vi "HTL_ErrorHandler.vi"(6 "error in":errorcluster) -> (0 "error out":errorcluster, 3 "All-Quit":bool)   [LabVIEW 2020]
doc: "Resets the CCD camera controller and initializes it with Setup String. The default Setup String is \"ldb,1,16,u,0,225,25,b,1,15;sdu,0,1024,1024;cl0;omrm;sron\". \nError, if no -1, is set as 0 if a serial poll detects an error (bit 15 in status bit set)\n\nSet the CCD Setup String Global variable after the command is complete."
uses:
  <vilib>/Utility/error.llb/DialogType.ctl
  Globals and TypeDefs/Type Definitions.llb/3 way Status.ctl
  Globals and TypeDefs/gDetector.vi
  Globals and TypeDefs/gSpectrometer.vi
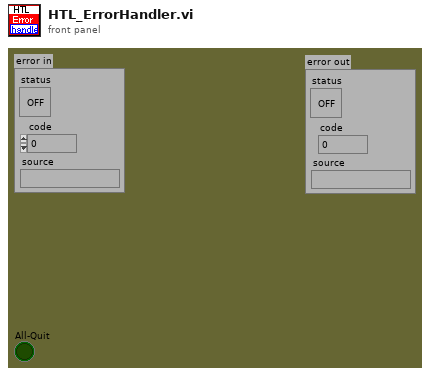
[diagram p1: front panel]
types:
  T1 = typedef "DialogType.ctl" = u16
  T2 = typedef "Error Categories.ctt" = enum8{"General", "CCD-256x1024", "CCD-1340x400", "InGaAs PDA", "McPherson 2075", "Magnetic Field", "Temperature Control", "Other"}
  T3 = enum16{"Left Button", "Center Button", "Right Button", "Window Close"}
  T4 = typedef "3 way Status.ctl" = u8
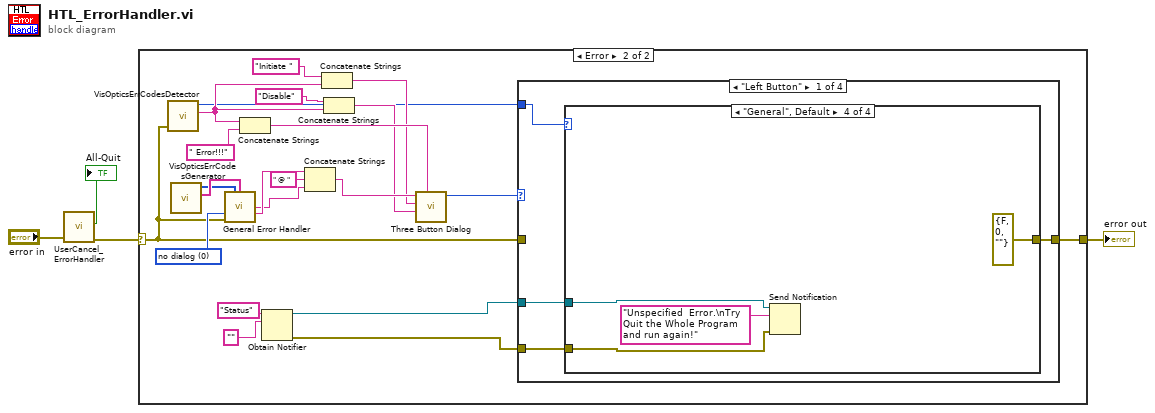
[diagram p0: block diagram]
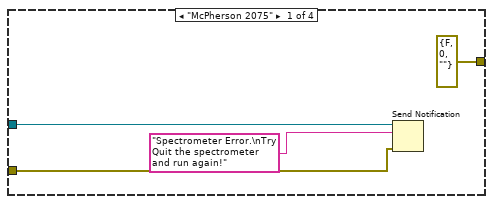
[diagram p3: hidden frame]
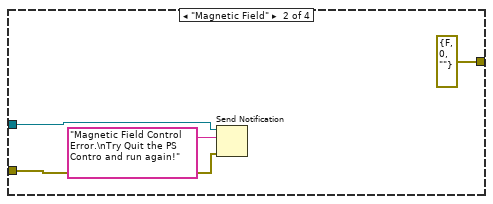
[diagram p4: hidden frame]
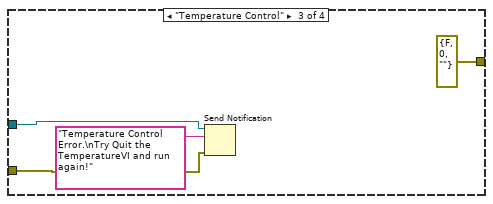
[diagram p5: hidden frame]
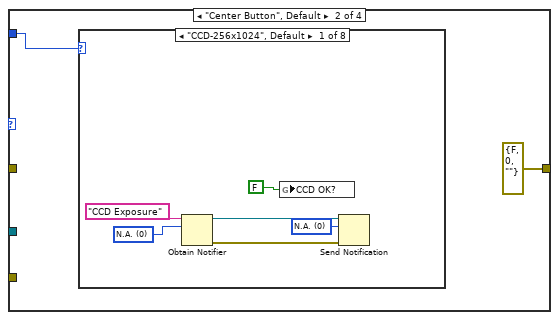
[diagram p6: hidden frame]
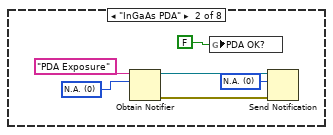
[diagram p7: hidden frame]
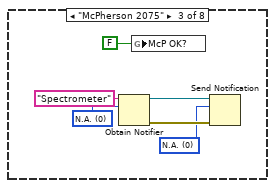
[diagram p8: hidden frame]
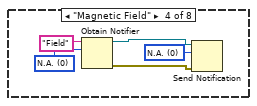
[diagram p9: hidden frame]
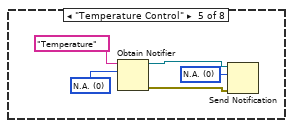
[diagram p10: hidden frame]
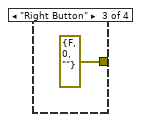
[diagram p14: hidden frame]
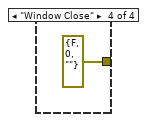
[diagram p15: hidden frame]
diagram:
  n1 = call "UserCancel_ErrorHandler.vi"("error in"="error in") -> ("error out"=w3:errorcluster, "All-Quit"=→"All-Quit":bool)  [unwired: 5 in, 1 out]
  n2 = case shown="Error" w3 {
    selector: w3 -> [w5 w22]
    tunnel: [w5 w23] -> w4
    frame No Error {
    }
    frame Error {
      w25 = T1 0 items=["no dialog", "OK message", "continue or stop message", "OK message + warnings", "continue/stop + warnings"] ("type of dialog (OK msg:1)")
      n3 = call "VisOpticsErrCodesDetector.vi"("error in"=w22) -> ("NHMFL Visible Optics Error Category"=w10:T2, "Error Category text"=w12:string)  [unwired: 2 in, 2 out]
      n4 = call "VisOpticsErrCodesGenerator.vi"() -> ("user-defined descriptions"=w27:string[], "user-defined codes"=w26:i32[])  [unwired: 3 in, 4 out]
      n5 = call <vilib>:"General Error Handler.vi"("[user-defined codes]"=w26, "[user-defined descriptions]"=w27, "type of dialog (OK msg:1)"=w25, "error in (no error)"=w22) -> ("source out"=w17:string, "message"=w19:string)  [unwired: 7 in, 3 out]
      n6 = Concatenate Strings(w12, " Error!!!" ("string")) -> (w20:string)
      n7 = Obtain Notifier(name (unnamed)="Status", notification data type="" ("Status")) -> (notifier out=w7:refnum<notifier>, error out=w6:errorcluster)  [unwired: 2 in, 1 out]
      n8 = Concatenate Strings(w19, " @ " ("string"), w17) -> (w16:string)
      n9 = Concatenate Strings("Initiate " ("Left Button Text (\"Yes\")"), w12) -> (w14:string)
      n10 = Concatenate Strings("Disable" ("Center Button Text (\"No\")"), w12) -> (w11:string)
      n11 = call <vilib>:"Three Button Dialog.vi"("Window Title (\"\")"=w20, "Center Button Text (\"No\")"=w11, "Left Button Text (\"Yes\")"=w14, "message"=w16) -> ("Which Button?"=w24:T3)  [unwired: 7 in]
      n12 = case shown="\"Left Button\"" w24 {
        tunnel: [w31 errorcluster {"status"=FALSE, "code"=0, "source"=""} ("error IO") errorcluster {"status"=FALSE, "code"=0, "source"=""} ("error IO") errorcluster {"status"=FALSE, "code"=0, "source"=""} ("error IO")] -> w23
        tunnel: w22 -> [_ _ _ _]
        tunnel: w10 -> [w30 w48 _ _]
        tunnel: w7 -> [w29 _ _ _]
        tunnel: w6 -> [w28 _ _ _]
        frame "Left Button" {
          n13 = case shown="\"General\", Default" w30 {
            tunnel: [errorcluster {"status"=FALSE, "code"=0, "source"=""} ("error IO") errorcluster {"status"=FALSE, "code"=0, "source"=""} ("error IO") errorcluster {"status"=FALSE, "code"=0, "source"=""} ("error IO") errorcluster {"status"=FALSE, "code"=0, "source"=""} ("error IO")] -> w31
            tunnel: w29 -> [w34 w37 w41 w45]
            tunnel: w28 -> [w33 w36 w40 w44]
            frame "McPherson 2075" {
              n14 = Send Notification(notification="Spectrometer Error.\nTry Quit the spectrometer and run again!", notifier=w34, error in (no error)=w33) -> ()  [unwired: 2 out]
            }
            frame "Magnetic Field" {
              n15 = Send Notification(notification="Magnetic Field Control Error.\nTry Quit the PS Contro and run again!", notifier=w37, error in (no error)=w36) -> ()  [unwired: 2 out]
            }
            frame "Temperature Control" {
              n16 = Send Notification(notification="Temperature Control Error.\nTry Quit the TemperatureVI and run again!", notifier=w41, error in (no error)=w40) -> ()  [unwired: 2 out]
            }
            frame "General", Default {
              n17 = Send Notification(notification="Unspecified  Error.\nTry Quit the Whole Program and run again!", notifier=w45, error in (no error)=w44) -> ()  [unwired: 2 out]
            }
          }
        }
        frame "Center Button", Default {
          n18 = case shown="\"CCD-256x1024\", Default" w48 {
            frame "CCD-256x1024", Default {
              w51 = T4 0 items=["N.A.", "OK", "Busy", "Done"] ("notification")
              w52 = T4 0 items=["N.A.", "OK", "Busy", "Done"] ("H(T)")
              n19 = Obtain Notifier(name (unnamed)="CCD Exposure", notification data type=w52) -> (notifier out=w54:refnum<notifier>, error out=w53:errorcluster)  [unwired: 2 in, 1 out]
              n20 = global write "gDetector.vi" "CCD OK?"(FALSE ("CCD OK?")) -> ()
              n21 = Send Notification(notification=w51, notifier=w54, error in (no error)=w53) -> ()  [unwired: 2 out]
            }
            frame "InGaAs PDA" {
              w57 = T4 0 items=["N.A.", "OK", "Busy", "Done"] ("notification")
              w60 = T4 0 items=["N.A.", "OK", "Busy", "Done"] ("H(T)")
              n22 = Obtain Notifier(name (unnamed)="PDA Exposure", notification data type=w60) -> (notifier out=w59:refnum<notifier>, error out=w58:errorcluster)  [unwired: 2 in, 1 out]
              n23 = global write "gDetector.vi" "PDA OK?"(FALSE ("CCD OK?")) -> ()
              n24 = Send Notification(notification=w57, notifier=w59, error in (no error)=w58) -> ()  [unwired: 2 out]
            }
            frame "McPherson 2075" {
              w63 = T4 0 items=["N.A.", "OK", "Busy", "Done"] ("notification")
              w66 = T4 0 items=["N.A.", "OK", "Busy", "Done"] ("Saving")
              n25 = Obtain Notifier(name (unnamed)="Spectrometer", notification data type=w66) -> (notifier out=w65:refnum<notifier>, error out=w64:errorcluster)  [unwired: 2 in, 1 out]
              n26 = global write "gSpectrometer.vi" "McP OK?"(FALSE ("McP OK?")) -> ()
              n27 = Send Notification(notification=w63, notifier=w65, error in (no error)=w64) -> ()  [unwired: 2 out]
            }
            frame "Magnetic Field" {
              w70 = T4 0 items=["N.A.", "OK", "Busy", "Done"] ("notification")
              w71 = T4 0 items=["N.A.", "OK", "Busy", "Done"] ("Saving")
              n28 = Obtain Notifier(name (unnamed)="Field", notification data type=w71) -> (notifier out=w69:refnum<notifier>, error out=w68:errorcluster)  [unwired: 2 in, 1 out]
              n29 = Send Notification(notification=w70, notifier=w69, error in (no error)=w68) -> ()  [unwired: 2 out]
            }
            frame "Temperature Control" {
              w75 = T4 0 items=["N.A.", "OK", "Busy", "Done"] ("notification")
              w76 = T4 0 items=["N.A.", "OK", "Busy", "Done"] ("Saving")
              n30 = Obtain Notifier(name (unnamed)="Temperature", notification data type=w76) -> (notifier out=w74:refnum<notifier>, error out=w73:errorcluster)  [unwired: 2 in, 1 out]
              n31 = Send Notification(notification=w75, notifier=w74, error in (no error)=w73) -> ()  [unwired: 2 out]
            }
            frame "Other" {
            }
            frame "CCD-1340x400" {
            }
            frame "General" {
            }
          }
        }
        frame "Right Button" {
        }
        frame "Window Close" {
        }
      }
    }
  }
  "error out" <- w4
